vi "Dictionary Filter by Word.vi"(10 "Words_Ref in":refnum<vi>[](array[refnum]), 11 "Dictionary in":string[](array[string])) -> (3 "Dictionary out":string[](array[string]))   [LabVIEW 2015]
uses:
  TypeDef/Color.ctl
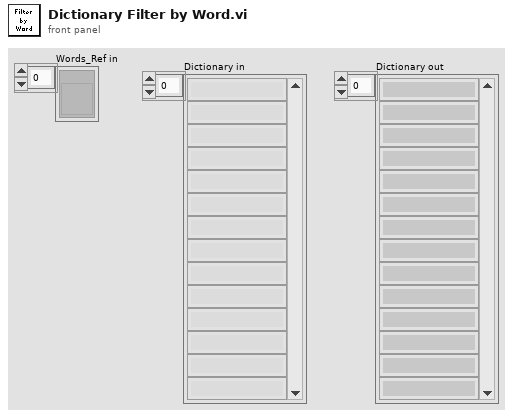
[diagram p1: front panel]
types:
  T1 = typedef "Color.ctl" = u32
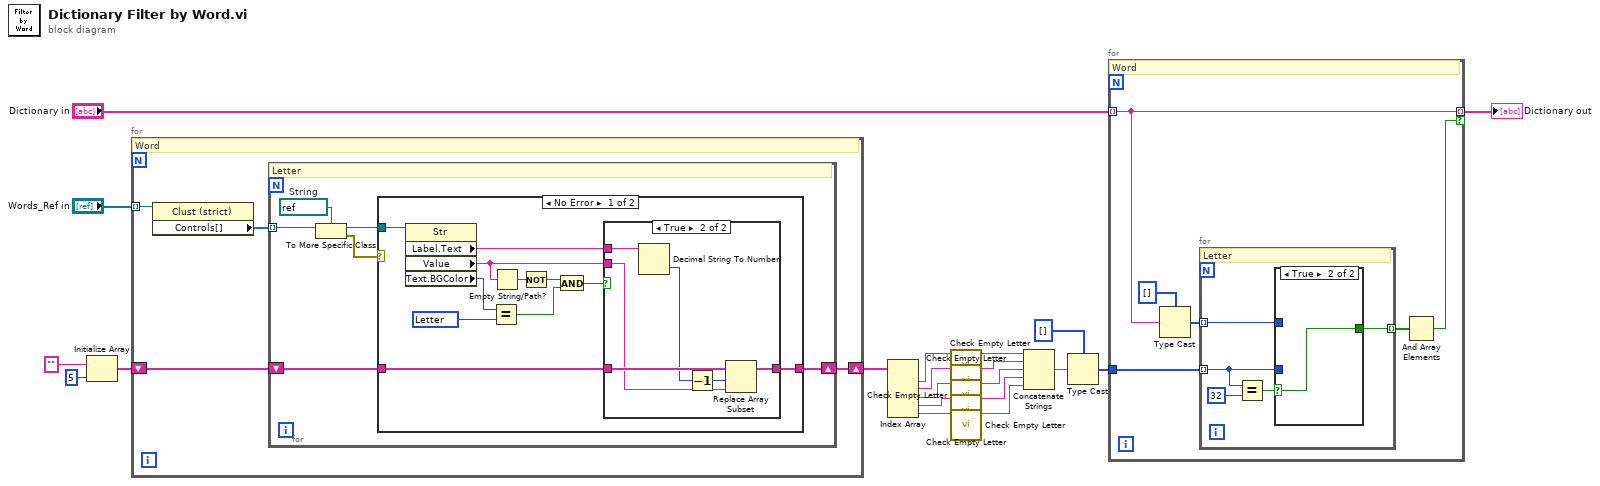
[diagram p0: block diagram]
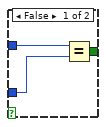
[diagram p4: hidden frame]
diagram:
  n1 = Initialize Array("", 5 ("dimension size")) -> (w7:string[])
  n2 = for {
    tunnel: "Words_Ref in" -> [w23] mode=indexing
    shift-right: [w21] -> w6
    shift-left: w7 -> [w22]
    # "Word"
    n3 = property class="Clust (strict)"(reference=w23) -> ("Controls[]"=w24:refnum<vi>[])  [unwired: 1 in, 2 out]
    n4 = for {
      tunnel: w24 -> [w28] mode=indexing
      shift-right: [w29] -> w21
      shift-left: w22 -> [w30]
      w26 = refnum<vi> refnum  # String
      # "Letter"
      n5 = To More Specific Class(target class=w26, reference=w28) -> (specific class reference=w27:refnum<vi>, error out=w25:errorcluster)  [unwired: 1 in]
      n6 = case shown="No Error" w25 {
        tunnel: w30 -> [w40 w49]
        tunnel: [w39 w49] -> w29
        tunnel: w27 -> [w38 _]
        frame No Error {
          w35 = T1 16774186 items=["Free"=9567230, "Letter"=16774186, "Any"=16448250, "Exclude"=12369084] ("Color")
          n7 = property class="Str"(reference=w38) -> ("Label.Text"=w41:string, "Value"=w31:string, "Text.BGColor"=w36:u32)  [unwired: 1 in, 2 out]
          n8 = Equal?(x=w36, y=w35) -> (x = y?=w33:bool)
          n9 = Empty String/Path?(string/path=w31) -> (empty?=w37:bool)
          n10 = Not(x=w37) -> (.not. x?=w34:bool)
          n11 = And(x=w34, y=w33) -> (x .and. y?=w32:bool)
          n12 = case shown="True" w32 {
            tunnel: w41 -> [_ w48]
            tunnel: w40 -> [w42 w47]
            tunnel: [w42 w46] -> w39
            tunnel: w31 -> [_ w43]
            frame False {
            }
            frame True {
              n13 = Decimal String To Number(string=w48) -> (number=w45:i32)  [unwired: 2 in, 1 out]
              n14 = Decrement(x=w45) -> (x-1=w44:i32)
              n15 = Replace Array Subset(array=w47, new element=w43, index=w44) -> (w46:string[])
            }
          }
        }
        frame Error {
        }
      }
    }
  }
  n16 = Index Array(array=w6) -> (element #1=w5:string, element #2=w4:string, element #3=w3:string, element #4=w2:string, element #5=w1:string)  [unwired: 5 in]
  n17 = call "Check Empty Letter.vi"("Letter in"=w5) -> ("Letter Out"=w17:string)  [unwired: 10 in]
  n18 = call "Check Empty Letter.vi"("Letter in"=w4) -> ("Letter Out"=w16:string)  [unwired: 10 in]
  n19 = call "Check Empty Letter.vi"("Letter in"=w3) -> ("Letter Out"=w15:string)  [unwired: 10 in]
  n20 = call "Check Empty Letter.vi"("Letter in"=w2) -> ("Letter Out"=w14:string)  [unwired: 10 in]
  n21 = call "Check Empty Letter.vi"("Letter in"=w1) -> ("Letter Out"=w13:string)  [unwired: 10 in]
  n22 = Concatenate Strings(w17, w16, w15, w14, w13) -> (w20:string)
  n23 = Type Cast(type=u8[] [], x=w20) -> (*(type *) &x=w18:u8[])
  n24 = for {
    tunnel: w18 -> [w55]
    tunnel: "Dictionary in" -> [w52] mode=indexing
    tunnel: [w52] -> w11 mode=indexing if=w50
    # "Word"
    n25 = Type Cast(type=u8[] [], x=w52) -> (*(type *) &x=w54:u8[])
    n26 = for {
      tunnel: w55 -> [w56] mode=indexing
      tunnel: w54 -> [w57] mode=indexing
      tunnel: [w58] -> w51 mode=indexing
      # "Letter"
      n27 = Equal?(x=w56, y=u8 32) -> (x = y?=w59:bool)
      n28 = case shown="True" w59 {
        selector: w59 -> [_ w64]
        tunnel: [w61 w64] -> w58
        tunnel: w57 -> [w63 _]
        tunnel: w56 -> [w62 _]
        frame False {
          n29 = Equal?(x=w63, y=w62) -> (x = y?=w61:bool)
        }
        frame True {
        }
      }
    }
    n30 = And Array Elements(Boolean array=w51) -> (logical AND=w50:bool)
  }
  "Dictionary out" <- w11
